vi "Module Name--constant.vi"() -> (3 "Module Name":string)   [LabVIEW 2025, in "N4L_PSM3750_Interface.lvlib"]
doc: "Return the name of the module that owns this VI. \n_____\nBased on Delacor QMH Project Template 3.1.0.34."
uses:
  N4L_PSM3750_Interface.lvlib
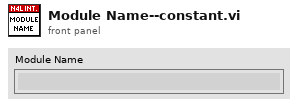
[diagram p1: front panel]
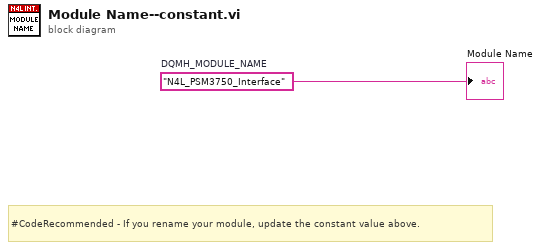
[diagram p0: block diagram]
diagram:
  w1 = "N4L_PSM3750_Interface"  # DQMH_MODULE_NAME
  # "#CodeRecommended - If you rename your module, update the constant value above."
  "Module Name" <- w1
